vi "STICK_house.vi"() -> ()   [LabVIEW 2014]
panel:
  out "On/Off":bool
  out "Error out":errorcluster
  out "P1":T1
  out "P2":T2
  out "Device ID":string
  in  "VISA resource name":refnum<visa-resource-name>
  out "Error":bool
  in  "Temp max":dbl=15.0
  in  "Temp min":dbl=-20.0
  in  "Thermostat ON/OFF":bool=TRUE
  out "Happiness [%]":dbl(slide) scale=0.0..100.0
  out "Status":string="Water frozen!"
  out "Thermostat [°C]":dbl=20.0
  out "Outdoor temp":dbl(slide) scale=-20.0..40.0
  out "Time":timestamp format="%<%H:%M>T"
  out "Heater temp":dbl(knob) max=60.0 scale=0.0..100.0
  out "Room temp":dbl(slide) scale=0.0..40.0
  out "Room [°C]":dbl format="%#_3g"
  out "Heater":bool
  in  "Thermostat [°C]":dbl=20.0 min=0.0 max=100.0
  in  "Heater temp [°C]":dbl=50.0 min=0.0 max=80.0 format="%#_2g"
  in  "T_room_0 [°C]":dbl=15.0 min=-40.0 max=100.0
  out "Waveform Chart":T3(graph)
  in  "Stop Button":bool
  # "System values"
  # "Thermostat"
  # "Boiler"
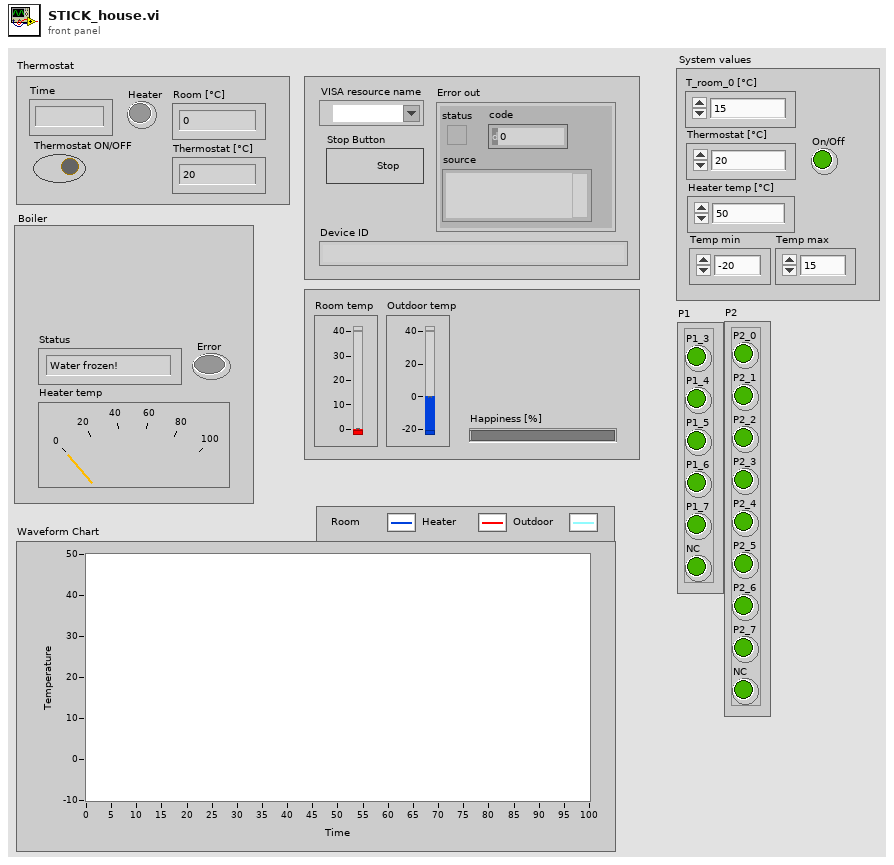
[diagram p1: front panel]
types:
  T1 = cluster{"P1_0":bool, "P1_1":bool, "P1_2":bool, "P1_3":bool, "P1_4":bool, "P1_5":bool, "P1_6":bool, "P1_7":bool, "NC":bool}
  T2 = cluster{"P2_0":bool, "P2_1":bool, "P2_2":bool, "P2_3":bool, "P2_4":bool, "P2_5":bool, "P2_6":bool, "P2_7":bool, "NC":bool}
  T3 = cluster{"T_room":dbl, "T_heater":dbl, "temp out":dbl}
  T4 = cluster{"T_room":dbl, "T_heater":dbl, "temp out":dbl}[]
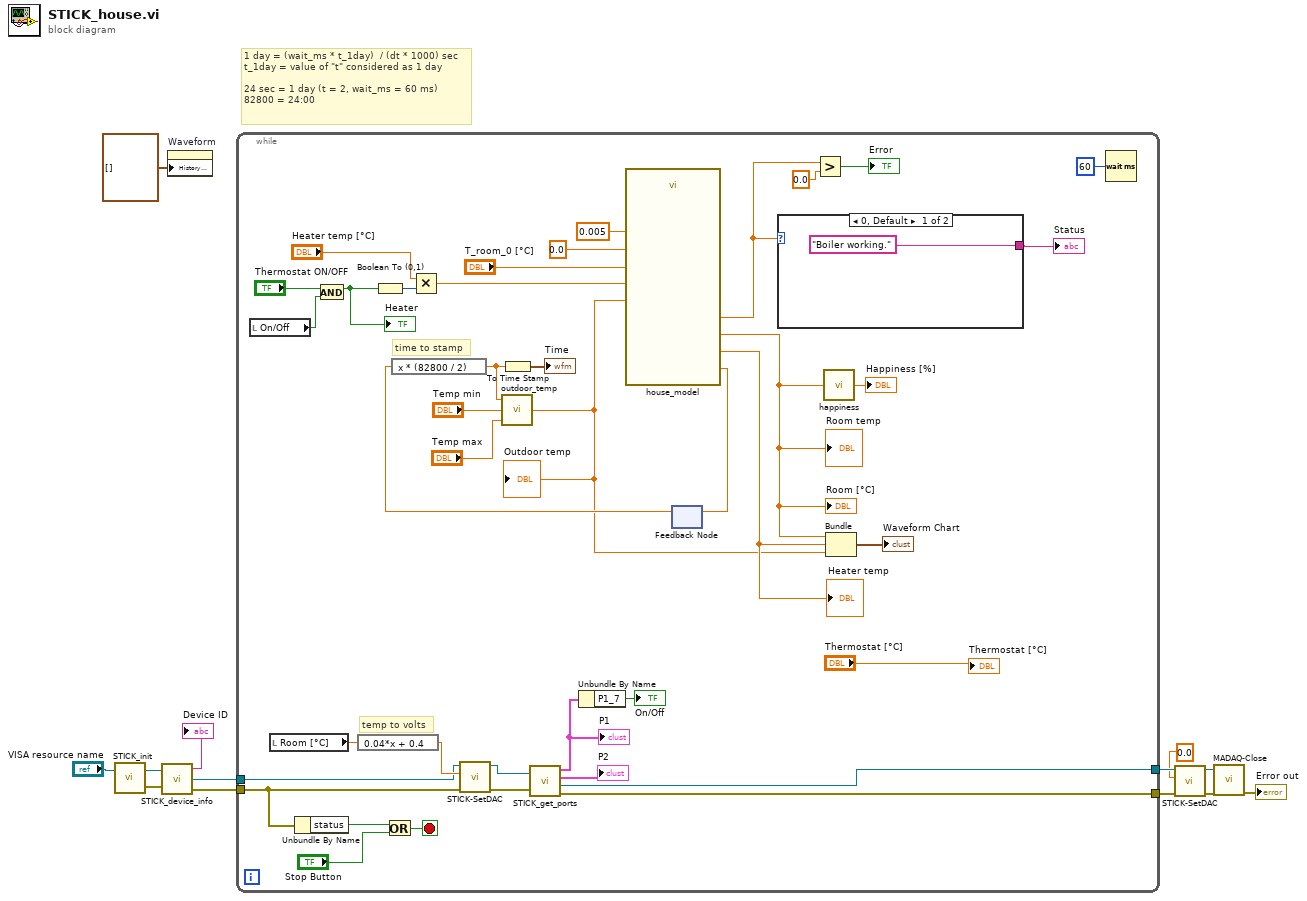
[diagram p0: block diagram]
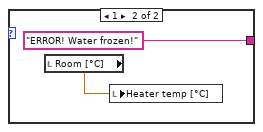
[diagram p2: hidden frame]
diagram:
  # "1 day = (wait_ms * t_1day)  / (dt * 1000) sec\nt_1day = value of \"t\" considered as 1 day\n\n24 sec = 1 day (t = 2, wait_ms = 60 ms)\n82800 = 24:00"
  n1 = call "STICK_init.vi"("VISA Refnum in"="VISA resource name") -> ("error out"=w11:errorcluster, "VISA Refnum out"=w10:refnum<visa-resource-name>)  [unwired: 1 in]
  n2 = call "STICK_device_info.vi"("VISA Refnum in"=w10, "error in (no error)"=w11) -> ("read buffer"=→"Device ID":string, "VISA Refnum out"=w1:refnum<visa-resource-name>, "error out"=w2:errorcluster)
  n3 = property on="Waveform" class="WFChart (strict)"("History Data"=T4 []) -> ()  [unwired: 2 in, 2 out]
  n4 = while {
    tunnel: [w22] -> w5
    tunnel: [w21] -> w3
    tunnel: w2 -> [w19]
    tunnel: w1 -> [w20]
    stop <- w26 stop-if-true
    # "time to stamp"
    # "temp to volts"
    n5 = local read "On/Off"() -> (w15:bool)
    n6 = local read "Room [°C]"() -> (w17:dbl)
    n7 = Unbundle By Name(w19) -> ("status"=w18:bool)
    n8 = And(x="Thermostat ON/OFF", y=w15) -> (x .and. y?=w33:bool)
    "Heater" <- w33
    n9 = expression code="0.04*x + 0.4"(w17) -> (w27:dbl)
    n10 = Boolean To (0,1)(Boolean=w33) -> (0, 1=w52:i16)
    n11 = Or(x=w18, y="Stop Button") -> (x .or. y?=w26:bool)
    n12 = Multiply(x="Heater temp [°C]", y=w52) -> (x*y=w51:dbl)
    n13 = call "STICK-SetDAC.vi"("error in (no error)"=w19, "IDA 0 [V]"=w27, "VISA resource name"=w20) -> ("error out"=w24:errorcluster, "VISA resource name out"=w23:refnum<visa-resource-name>)  [unwired: 3 in]
    n14 = call "STICK_get_ports.vi"("error in (no error)"=w24, "VISA Refnum in"=w23) -> ("error out"=w21:errorcluster, "VISA Refnum out"=w22:refnum<visa-resource-name>, "P2"=→"P2":T2, "P1"=w29:T1)  [unwired: 1 out]
    "P1" <- w29
    n15 = Unbundle By Name(w29) -> ("P1_7"=→"On/Off":bool)
    n16 = feedback #1() -> (w39:dbl)  [unwired: 1 in]
    n17 = expression code="x * (82800 / 2)"(w39) -> (w49:dbl)
    n18 = call "outdoor_temp.vi"("temp max"="Temp max", "temp min"="Temp min", "time in"=w49) -> ("temp out"=w36:dbl)
    "Outdoor temp" <- w36
    n19 = To Time Stamp(1:w49) -> (0:→"Time":timestamp)
    n20 = call "house_model.vi"("T_out"=w36, "dt"=0.005, "t_0"=0.0 ("t"), "T_room_0"="T_room_0 [°C]", "heat_level"=w51) -> ("T_room"=w31:dbl, "error_code"=w44:dbl, "t"=w37:dbl, "T_heater"=w41:dbl)  [unwired: 5 in, 2 out]
    "Room [°C]" <- w31
    "Room temp" <- w31
    "Heater temp" <- w41
    n21 = feedback-in #1(w37) -> ()
    n22 = case shown="0, Default" w44 {
      tunnel: ["Boiler working." "ERROR! Water frozen!"] -> w32
      frame 0, Default {
      }
      frame 1 {
        n23 = local read "Room [°C]"() -> (w55:dbl)
        n24 = local write "Heater temp [°C]"(w55) -> ()
      }
    }
    "Status" <- w32
    n25 = Greater?(x=w44, y=0.0) -> (0:→"Error":bool)
    n26 = call "happiness.vi"("T_room"=w31) -> ("Happiness [%]"=→"Happiness [%]":dbl)
    n27 = Bundle("T_room"=w31, "T_heater"=w41, "temp out"=w36) -> (→"Waveform Chart":T3)  [unwired: 1 in]
    n28 = Wait (ms)(milliseconds to wait=u32 60) -> ()  [unwired: 1 out]
    "Thermostat [°C]" <- "Thermostat [°C]"
  }
  n29 = call "STICK-SetDAC.vi"("error in (no error)"=w3, "IDA 0 [V]"=0.0 ("DAC  1 [V]"), "VISA resource name"=w5) -> ("error out"=w7:errorcluster, "VISA resource name out"=w6:refnum<visa-resource-name>)  [unwired: 3 in]
  n30 = call "MADAQ-Close.vi"("error in (no error)"=w7, "VISA resource name"=w6) -> ("error out"=→"Error out":errorcluster)  [unwired: 4 in, 1 out]
